vi "provide_OME_data.vi"(6 "image ID":string, 8 "error in (no error)":errorcluster, 9 "structuredAttribute string in":string, 10 "OME element in":refnum<class "XMLElement.lvclass">, 11 "DL090603DAQmxOnOffDetector in":refnum<class "DetectorDL090603DAQmxOnOff.lvclass">) -> (0 "error out":errorcluster, 1 "structuredAttribute string out":string, 2 "OME element out":refnum<class "XMLElement.lvclass">, 3 "DL090603DAQmxOnOffDetector out":refnum<class "DetectorDL090603DAQmxOnOff.lvclass">)   [LabVIEW 2010, in "DetectorDL090603DAQmxOnOff.lvclass"]
uses:
  DetectorDL090603DAQmxOnOff.lvclass
  common/classes/XMLElement/XMLElement/XMLElement.lvclass
  GenericDetector/GenericDetector/GenericDetector.lvclass
  DetectorDL090603DAQmxOnOff.lvclass/DetectorDL090603DAQmxOnOff.ctl
  common/classes/ErrorController/ErrorController/class_data.vi
  Instrument/GenericInstrument/GenericInstrument/GenericInstrument.lvclass
  common/classes/ErrorController/ErrorController/ErrorController.lvclass
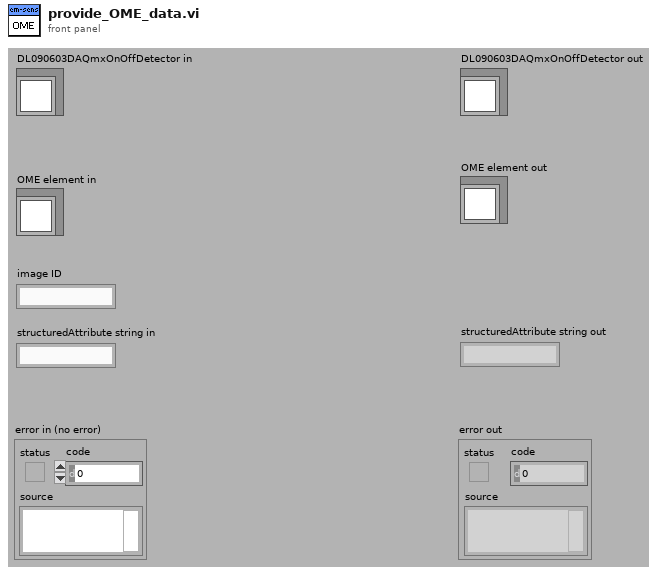
[diagram p1: front panel]
types:
  T1 = typedef "GenericDetector.lvclass/type_enum.ctl" = enum16{"CCD", "IntensifiedCCD", "AnalogVideo", "PMT", "Photodiode", "Spectoscropy", "LifetimeImaging", "CorrelationSpectroscopy", "FTIR", "EM-CCD", "APD", "CMOS", "Unknown"}
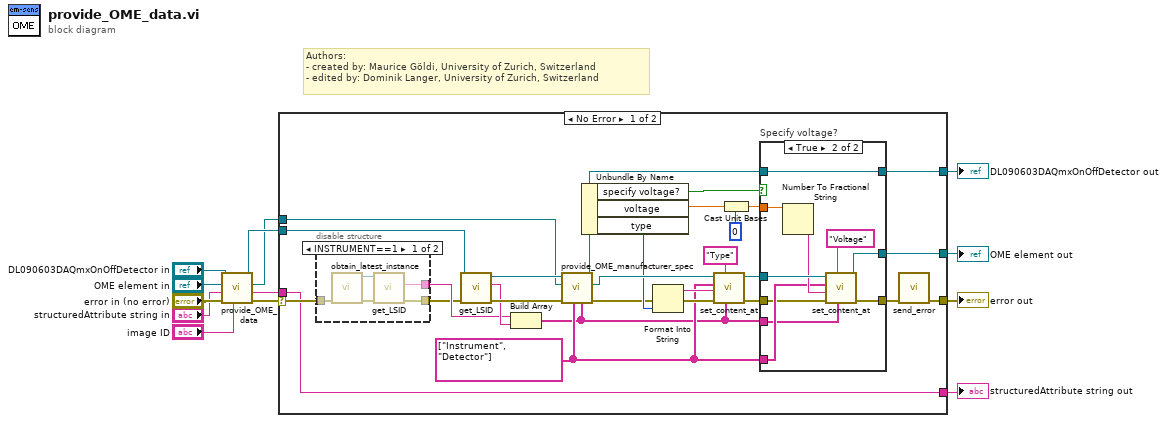
[diagram p0: block diagram]
diagram:
  # "Authors: \n- created by: Maurice Göldi, University of Zurich, Switzerland\n- edited by: Dominik Langer, University of Zurich, Switzerland"
  n1 = call-parent "provide_OME_data.vi"("image ID"="image ID", "error in (no error)"="error in (no error)", "structuredAttribute string in"="structuredAttribute string in", "OME element in"="OME element in", "GenericPlugin in"="DL090603DAQmxOnOffDetector in") -> ("error out"=w10:errorcluster, "structuredAttribute string out"=w2:string, "OME element out"=w7:refnum<class "XMLElement.lvclass">, "GenericPlugin out"=w8:refnum<class "DetectorDL090603DAQmxOnOff.lvclass">)  [unwired: 3 in]
  n2 = case shown="No Error" w10 {
    selector: w10 -> [w26 w64]
    tunnel: [w23 w64] -> w13
    tunnel: w8 -> [w17 w63]
    tunnel: [w38 w62] -> w5
    tunnel: w7 -> [w15 w62]
    tunnel: [w36 w63] -> w12
    tunnel: w2 -> [w20 w61]
    tunnel: [w20 w61] -> w1
    frame No Error {
      w24 = string[] ["Instrument", "Detector"]
      n3 = disable-structure shown="INSTRUMENT==1" {
        disable-tunnel: w26 -> [w44 w47]
        disable-tunnel: [w43 w47] -> w27
        disable-tunnel: [w42 _] -> w28
        frame condition #0 {
          n4 = call "obtain_latest_instance.vi"("error in (no error)"=w44) -> ("error out"=w45:errorcluster, "microscope"=w46:refnum<class "GenericInstrument.lvclass">)  [unwired: 9 in]
          n5 = call-dynamic "get_LSID.vi"("error in (no error)"=w45, "GenericPlugin in"=w46) -> ("error out"=w43:errorcluster, "LSID (string)"=w42:string)  [unwired: 6 in, 2 out]
        }
        frame condition #1 (active) {
        }
      }
      n6 = call-dynamic "get_LSID.vi"("error in (no error)"=w27, "GenericPlugin in"=w17) -> ("error out"=w32:errorcluster, "LSID (string)"=w29:string, "GenericPlugin out"=w33:refnum<class "DetectorDL090603DAQmxOnOff.lvclass">)  [unwired: 6 in, 1 out]
      n7 = Build Array(w28, w29) -> (w21:string[])
      n8 = call-dynamic "provide_OME_manufacturer_spec.vi"("id chain"=w21, "key chain"=w24, "error in (no error)"=w32, "XMLElement in"=w15, "GenericPlugin in"=w33) -> ("error out"=w18:errorcluster, "XMLElement out"=w31:refnum<class "XMLElement.lvclass">, "GenericPlugin out"=w16:refnum<class "DetectorDL090603DAQmxOnOff.lvclass">)  [unwired: 4 in]
      n9 = Unbundle By Name(w16) -> ("specify voltage?"=w37:bool, "voltage"=w41:dbl[unit], "type"=w19:T1)
      n10 = Format Into String(error in=w18, w19) -> (resulting string=w34:string, error out=w30:errorcluster)  [unwired: 2 in]
      n11 = call "set_content_at.vi"("id chain"=w21, "attribute name"="Type", "error in (no error)"=w30, "content"=w34, "key chain"=w24, "Element in"=w31) -> ("error out"=w25:errorcluster, "Element out"=w14:refnum<class "XMLElement.lvclass">)  [unwired: 4 in]
      n12 = Cast Unit Bases(0:w41, 1:0) -> (2:w40:dbl)
      n13 = case "Specify voltage?" shown="True" w37 {
        tunnel: [w49 w57] -> w38
        tunnel: w14 -> [w49 w58]
        tunnel: w25 -> [w50 w51]
        tunnel: [w50 w59] -> w22
        tunnel: w40 -> [_ w60]
        tunnel: w16 -> [w48 w52]
        tunnel: [w48 w52] -> w36
        tunnel: w24 -> [_ w54]
        tunnel: w21 -> [_ w53]
        frame False {
        }
        frame True {
          n14 = Number To Fractional String(number=w60) -> (F-format string=w56:string)  [unwired: 3 in]
          n15 = call "set_content_at.vi"("id chain"=w53, "attribute name"="Voltage", "error in (no error)"=w51, "content"=w56, "key chain"=w54, "Element in"=w58) -> ("error out"=w59:errorcluster, "Element out"=w57:refnum<class "XMLElement.lvclass">)  [unwired: 4 in]
        }
      }
      n16 = call "send_error.vi"("error in (no error)"=w22) -> ("error out"=w23:errorcluster)  [unwired: 10 in]
    }
    frame Error {
    }
  }
  "error out" <- w13
  "DL090603DAQmxOnOffDetector out" <- w12
  "OME element out" <- w5
  "structuredAttribute string out" <- w1
